vi "Set Fill Volume Impl.vi"(8 "error in (no error)":errorcluster, 10 "Volume, uL":u16, 11 "Alltesta Autosampler in":refnum<class "Alltesta Autosampler.lvclass">) -> (0 "error out":errorcluster, 3 "Alltesta Autosampler out":refnum<class "Alltesta Autosampler.lvclass">)   [LabVIEW 2023, in "Alltesta Autosampler.lvlib" / "Alltesta Autosampler.lvclass"]
uses:
  Alltesta Autosampler.lvclass
  Alltesta Autosampler.lvclass/Alltesta Autosampler.ctl
  Alltesta Autosampler.lvlib
panel:
  out "Response":string
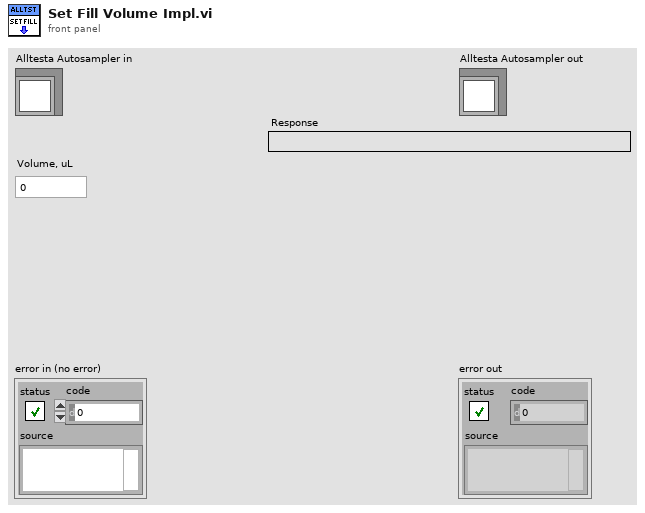
[diagram p1: front panel]
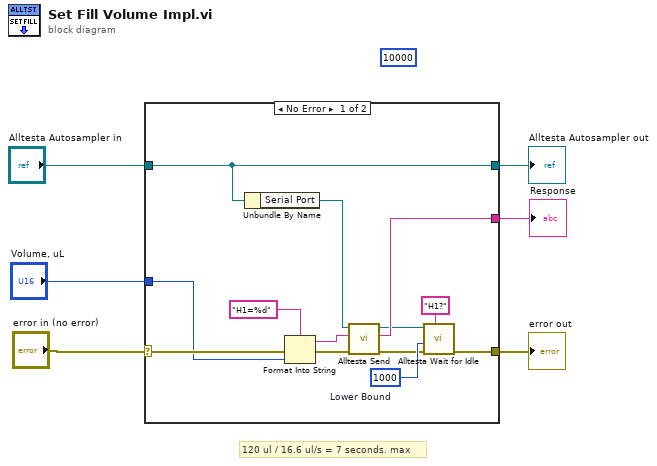
[diagram p0: block diagram]
diagram:
  (unwired) 10000 ("y")
  # "120 ul / 16.6 ul/s = 7 seconds. max"
  n1 = case shown="No Error" "error in (no error)" {
    selector: "error in (no error)" -> [w18 w21]
    tunnel: [w7 w21] -> w2
    tunnel: "Alltesta Autosampler in" -> [w14 w20]
    tunnel: [w14 w20] -> w3
    tunnel: "Volume, uL" -> [w13 _]
    tunnel: [w12 _] -> w1
    frame No Error {
      w10 = 1000  # Lower Bound
      n2 = Unbundle By Name(w14) -> ("Serial Port"=w19:refnum<visa-resource-name>)
      n3 = Format Into String(format string="H1=%d", error in=w18, w13) -> (resulting string=w16:string, error out=w17:errorcluster)  [unwired: 1 in]
      n4 = call "Alltesta Send.vi"("error in (no error)"=w17, "Command"=w16, "Serial Port in"=w19) -> ("error out"=w9:errorcluster, "Response"=w12:string, "Serial Port out"=w8:refnum<visa-resource-name>)  [unwired: 6 in]
      n5 = call "Alltesta Wait for Idle.vi"("Poll Command"="H1?", "error in (no error)"=w9, "Lower Bound"=w10, "Serial Port in"=w8) -> ("error out"=w7:errorcluster)  [unwired: 6 in, 1 out]
    }
    frame Error {
    }
  }
  "error out" <- w2
  "Alltesta Autosampler out" <- w3
  "Response" <- w1
